vi "基础17.vi"() -> ()   [LabVIEW 2014]
panel:
  in  "停止":bool
  in  "簇 2":T1 {"旋钮" scale=0.0..10.0; "滑动杆" scale=0.0..10.0}
  out "簇":T2 {"量表 2" scale=0.0..300.0; "量表" scale=0.0..300.0; "滑动杆" scale=0.0..100.0}
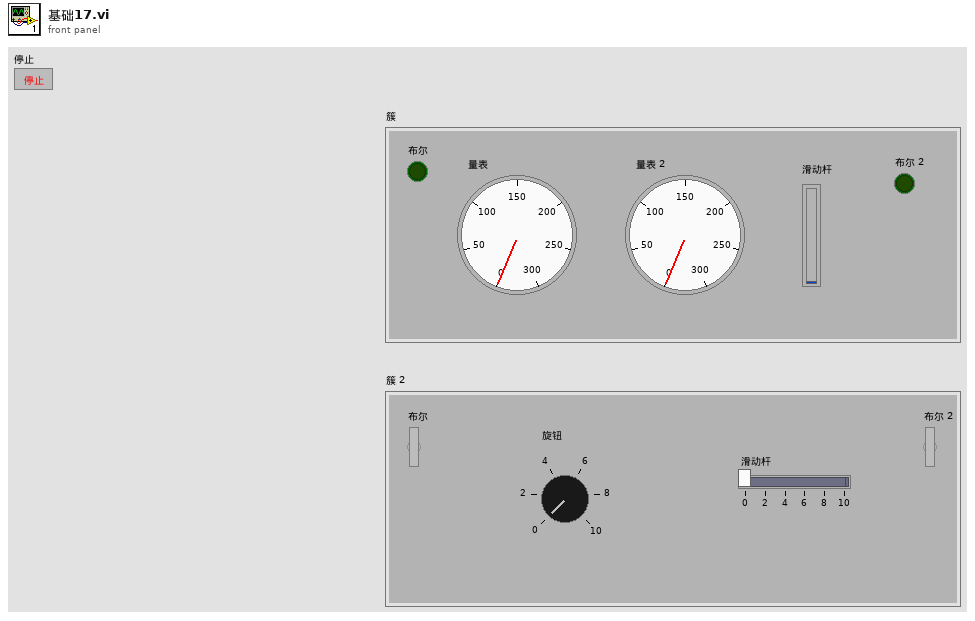
[diagram p1: front panel]
types:
  T1 = cluster{"布尔":bool, "布尔 2":bool, "滑动杆":dbl, "旋钮":dbl}
  T2 = cluster{"布尔":bool, "布尔 2":bool, "滑动杆":u8, "量表":dbl, "量表 2":dbl}
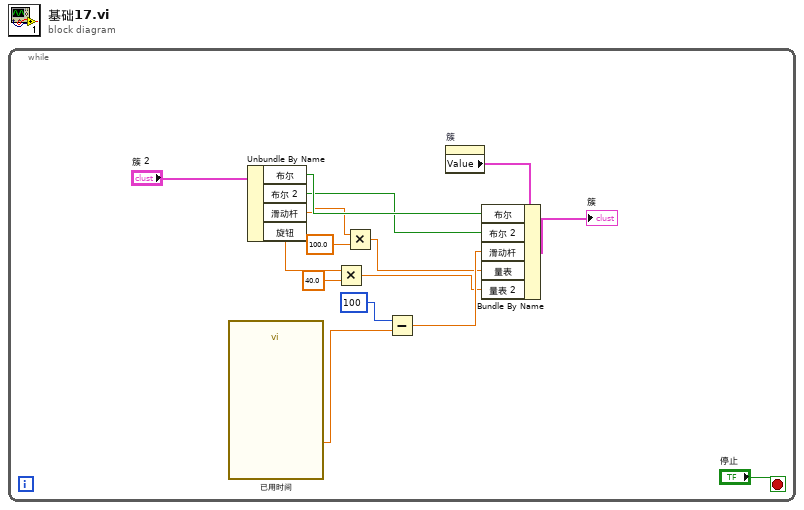
[diagram p0: block diagram]
diagram:
  n1 = while {
    stop <- "停止" stop-if-true
    n2 = call "已用时间"() -> ("Elapsed Time (s)"=w1:dbl)  [unwired: 12 in, 7 out]
    n3 = Unbundle By Name("簇 2") -> ("布尔"=w9:bool, "布尔 2"=w8:bool, "滑动杆"=w7:dbl, "旋钮"=w4:dbl)
    n4 = Multiply(x=w4, y=40.0) -> (x*y=w2:dbl)
    n5 = Multiply(x=w7, y=100.0) -> (x*y=w5:dbl)
    n6 = Subtract(x=100, y=w1) -> (x-y=w10:dbl)
    n7 = property on="簇" class="Clust (严格)"() -> ("Value"=w14:T2)  [unwired: 2 in, 2 out]
    n8 = Bundle By Name(cluster=w14, "布尔"=w9, "布尔 2"=w8, "滑动杆"=w10, "量表"=w5, "量表 2"=w2) -> (→"簇":T2)
  }
